vi "Example Graph - Reflectivity Callback.vi"(4 "Reflectivity":refnum<user-event>, 5 "Event Data":T1, 6 "Control Ref":refnum<k24>, 7 "Event Common Data":T2) -> ()   [LabVIEW 2010]
uses:
  C:/tf/play/labview/Tinkerforge.dll
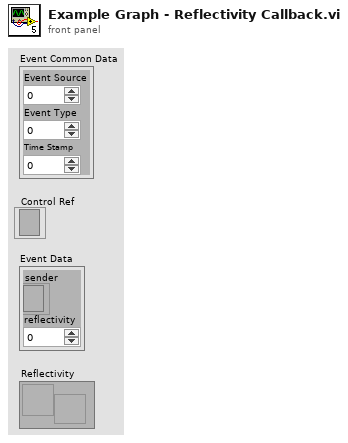
[diagram p1: front panel]
types:
  T1 = cluster{"sender":refnum<k24>, "reflectivity":i32}
  T2 = cluster{"Event Source":i32, "Event Type":u32, "Time Stamp":u32}
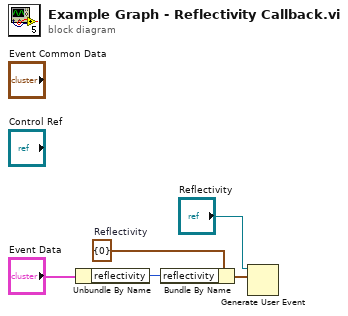
[diagram p0: block diagram]
diagram:
  w3 = cluster{"reflectivity":i32} {"reflectivity"=0}  # Reflectivity
  n1 = Unbundle By Name("Event Data") -> ("reflectivity"=w4:i32)
  n2 = Bundle By Name(cluster=w3, "reflectivity"=w4) -> (w2:cluster{"reflectivity":i32})
  n3 = Generate User Event(user event="Reflectivity", event data cluster=w2) -> ()  [unwired: 1 in, 2 out]
